vi "BuildHelpPath.vi"(1 "Help File Name":string="lvhelp.chm" caption="Name der Hilfe-Datei") -> (0 "Help File Path":path caption="Pfad der Hilfe-Datei")   [LabVIEW 2009]
doc: "Dieses VI fügt den angegebenen Dateinamen an das Hilfe-Verzeichnis an und gibt den vollständigen Pfad zurück. Wird kein Dateiname angegeben, wird die LabVIEW-Hilfe als Voreinstellung verwendet."
panel:
  # "Dieses VI fügt den angegebenen Dateinamen an das Hilfe-Verzeichnis an\n und gibt den vollständigen Pfad zurück. Wird kein Dateiname angegeben, wird die LabVIEW-Hilfe als Voreinstellung verwendet."
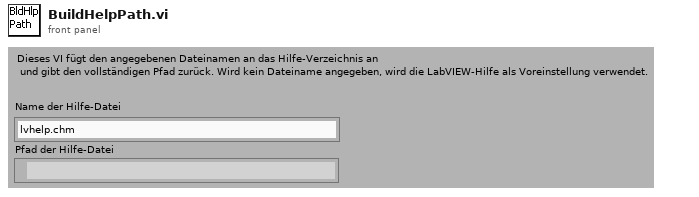
[diagram p1: front panel]
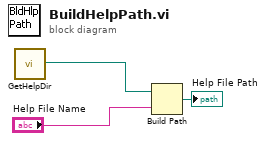
[diagram p0: block diagram]
diagram:
  n1 = call "GetHelpDir.vi"() -> ("help path"=w3:path)
  n2 = Build Path(base path=w3, name or relative path="Help File Name") -> (appended path=→"Help File Path":path)
